vi "nD Line Search (VI).vi"(5 "J":dbl[][](array[numeric]) format="%.2f", 6 "data":variant, 7 "F(X)":T1, 8 "TOLX":dbl=1e-07 format="%.2e", 9 "alpha":dbl=0.0001 format="%.2e", 10 "P":dbl[](array[numeric]) format="%.2f", 11 "X":dbl[](array[numeric]) format="%.2f") -> (0 "error":i32, 2 "index":u32, 3 "X (new)":dbl[](array[numeric]) format="%.2f")   [LabVIEW 2010, in "NI_Gmath.lvlib"]
uses:
  NI_Gmath.lvlib
  functionRefnum nD.ctl
  Real Dot Product.vi
  NI_AALBase.lvlib
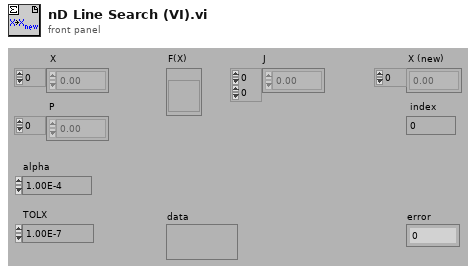
[diagram p1: front panel]
types:
  T1 = typedef "NI_Gmath.lvlib/functionRefnum nD.ctl" = refnum<vi>
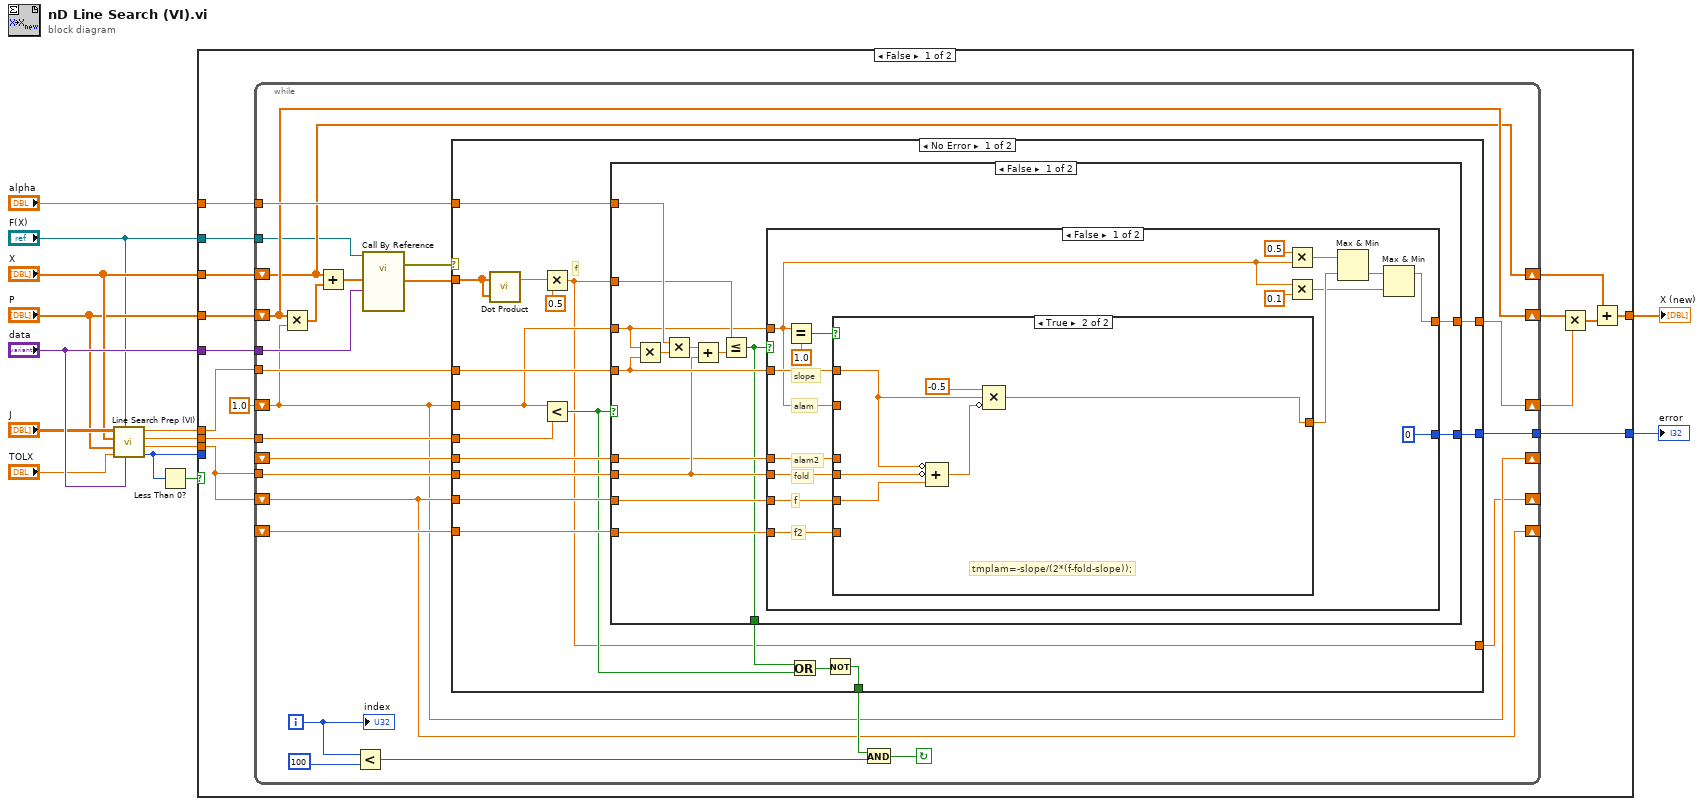
[diagram p0: block diagram]
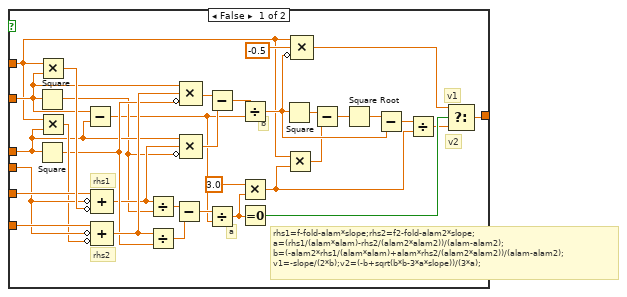
[diagram p2: hidden frame]
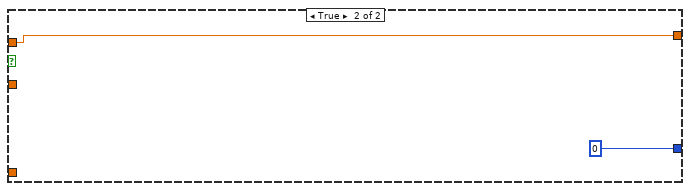
[diagram p3: hidden frame]
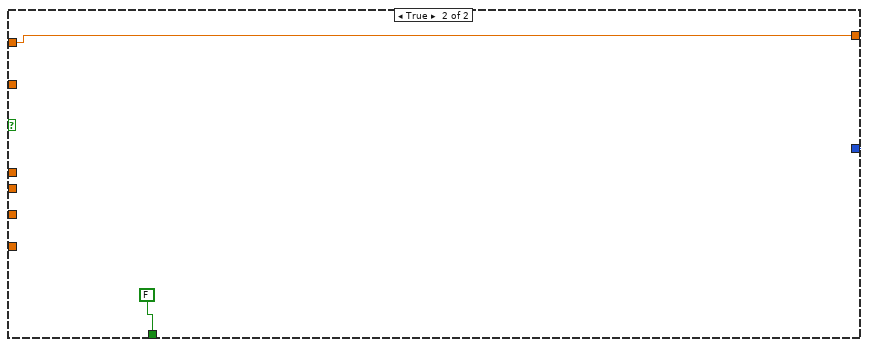
[diagram p4: hidden frame]
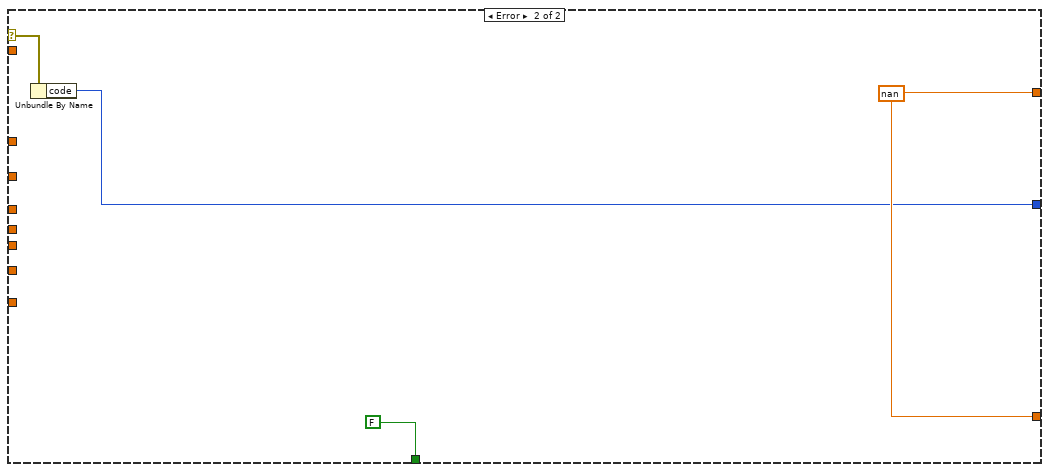
[diagram p5: hidden frame]
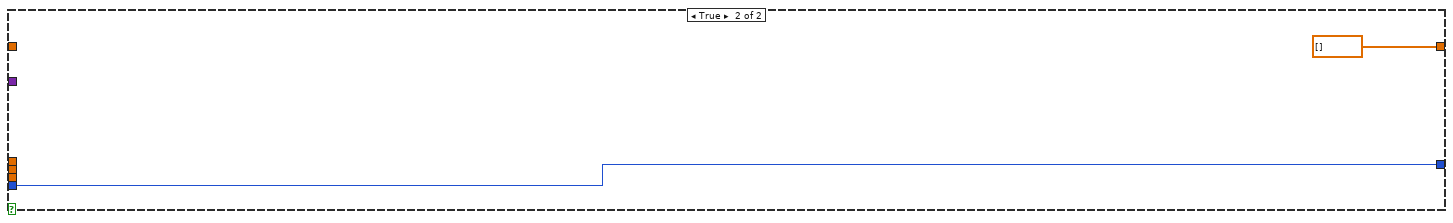
[diagram p6: hidden frame]
diagram:
  n1 = call "Line Search Prep (VI).vi"("data"="data", "F(X)"="F(X)", "TOLX"="TOLX", "P"="P", "X"="X", "J"="J") -> ("error"=w3:i32, "F(X)*F(X)"=w9:dbl, "tolerance"=w11:dbl, "X * Y"=w10:dbl)  [unwired: 2 out]
  n2 = Less Than 0?(x=w3) -> (x < 0?=w4:bool)
  n3 = case shown="False" w4 {
    tunnel: "data" -> [w29 _]
    tunnel: w11 -> [w27 _]
    tunnel: w10 -> [w26 _]
    tunnel: w9 -> [w25 _]
    tunnel: [w20 dbl[] []] -> w8
    tunnel: "alpha" -> [w19 _]
    tunnel: "X" -> [w18 _]
    tunnel: "P" -> [w17 _]
    tunnel: "F(X)" -> [w16 _]
    tunnel: w3 -> [_ w151]
    tunnel: [w15 w151] -> w2
    frame False {
      n4 = while {
        tunnel: w25 -> [w49]
        tunnel: w26 -> [w50]
        tunnel: w19 -> [w51]
        tunnel: w27 -> [w52]
        shift-left: _ -> [w48]
        shift-right: [w35] -> _
        shift-left: w25 -> [w35]
        shift-right: [w32] -> _
        shift-left: _ -> [w47]
        shift-right: [w34] -> _
        shift-left: 1.0 -> [w34]
        shift-right: [w43] -> w23
        shift-left: w17 -> [w46]
        shift-right: [w46] -> w22
        shift-left: w18 -> [w45]
        shift-right: [w45] -> w24
        tunnel: w16 -> [w38]
        tunnel: w29 -> [w37]
        tunnel: [w33] -> w15
        i -> [w44]
        stop <- w39 continue-if-true
        n5 = Multiply(x=w46, y=w34) -> (x*y=w53:dbl[])
        n6 = Add(x=w45, y=w53) -> (x+y=w31:dbl[])
        n7 = Less?(x=w44, y=100) -> (x < y?=w41:bool)
        n8 = call-by-ref "?"(reference=w38, "variant"=w37, "X"=w31) -> (error out=w30:errorcluster, "F(X)"=w36:dbl[])  [unwired: 4 in, 1 out]
        n9 = case shown="No Error" w30 {
          selector: w30 -> [_ w147]
          tunnel: w52 -> [w71 _]
          tunnel: w51 -> [w70 _]
          tunnel: w50 -> [w69 _]
          tunnel: w49 -> [w68 _]
          tunnel: w35 -> [w64 _]
          tunnel: w48 -> [w63 _]
          tunnel: w47 -> [w62 _]
          tunnel: [w59 w148] -> w43
          tunnel: [w58 FALSE] -> w40
          tunnel: w36 -> [w57 _]
          tunnel: w34 -> [w56 _]
          tunnel: [w55 w148] -> w32
          tunnel: [w54 w146] -> w33
          frame No Error {
            # "f"
            n10 = call-poly "Dot Product.vi"("Y Vector"=w57, "X Vector"=w57) -> ("X * Y"=w67:dbl)  [unwired: 1 out]
            n11 = Multiply(x=w67, y=0.5) -> (x*y=w55:dbl)
            n12 = Less?(x=w56, y=w71) -> (x < y?=w61:bool)
            n13 = case shown="False" w61 {
              tunnel: w70 -> [w85 _]
              tunnel: w56 -> [w80 w144]
              tunnel: w69 -> [w78 _]
              tunnel: w68 -> [w76 _]
              tunnel: w55 -> [w81 _]
              tunnel: [w73 FALSE] -> w65
              tunnel: [w79 w144] -> w59
              tunnel: w64 -> [w77 _]
              tunnel: w63 -> [w75 _]
              tunnel: w62 -> [w74 _]
              tunnel: [w72 0] -> w54
              frame False {
                n14 = Multiply(x=w80, y=w78) -> (x*y=w84:dbl)
                n15 = Multiply(x=w85, y=w84) -> (x*y=w83:dbl)
                n16 = Add(x=w83, y=w76) -> (x+y=w82:dbl)
                n17 = Less Or Equal?(x=w81, y=w82) -> (x <= y?=w73:bool)
                n18 = case shown="False" w73 {
                  tunnel: w80 -> [w89 w142]
                  tunnel: [w93 w142] -> w79
                  tunnel: w78 -> [w92 _]
                  tunnel: w77 -> [w91 _]
                  tunnel: w76 -> [w90 _]
                  tunnel: w75 -> [w88 _]
                  tunnel: w74 -> [w87 _]
                  tunnel: [0 0] -> w72
                  frame False {
                    # "f2"
                    # "f"
                    # "slope"
                    # "fold"
                    # "alam2"
                    # "alam"
                    n19 = Equal?(x=w89, y=1.0) -> (x = y?=w100:bool)
                    n20 = case shown="True" w100 {
                      tunnel: [w133 w138] -> w97
                      tunnel: w92 -> [w106 w135]
                      tunnel: w91 -> [w131 w137]
                      tunnel: w90 -> [w129 w136]
                      tunnel: w89 -> [w124 _]
                      tunnel: w88 -> [w130 _]
                      tunnel: w87 -> [w119 _]
                      frame False {
                        # "rhs1=f-fold-alam*slope;rhs2=f2-fold-alam2*slope;\na=(rhs1/(alam*alam)-rhs2/(alam2*alam2))/(alam-alam2);\nb=(-alam2*rhs1/(alam*alam)+alam*rhs2/(alam2*alam2))/(alam-alam2);\nv1=-slope/(2*b);v2=(-b+sqrt(b*b-3*a*slope))/(3*a);"
                        # "rhs2"
                        # "rhs1"
                        # "b"
                        # "v2"
                        # "v1"
                        # "a"
                        n21 = Square(x=w124) -> (x^2=w118:dbl)
                        n22 = Square(x=w119) -> (x^2=w122:dbl)
                        n23 = Multiply(x=w106, y=w124) -> (x*y=w132:dbl)
                        n24 = Multiply(x=w106, y=w119) -> (x*y=w128:dbl)
                        n25 = Subtract(x=w124, y=w119) -> (x-y=w115:dbl)
                        n26 = Compound Arithmetic op=ADD(w131, invert w129, invert w132) -> (w120:dbl)
                        n27 = Compound Arithmetic op=ADD(w130, invert w129, invert w128) -> (w123:dbl)
                        n28 = Divide(x=w120, y=w118) -> (x/y=w127:dbl)
                        n29 = Divide(x=w123, y=w122) -> (x/y=w126:dbl)
                        n30 = Subtract(x=w127, y=w126) -> (x-y=w125:dbl)
                        n31 = Compound Arithmetic op=MULTIPLY(w124, w123, invert w122) -> (w121:dbl)
                        n32 = Compound Arithmetic op=MULTIPLY(w119, w120, invert w118) -> (w117:dbl)
                        n33 = Subtract(x=w121, y=w117) -> (x-y=w116:dbl)
                        n34 = Divide(x=w125, y=w115) -> (x/y=w107:dbl)
                        n35 = Divide(x=w116, y=w115) -> (x/y=w109:dbl)
                        n36 = Multiply(x=3.0, y=w107) -> (x*y=w103:dbl)
                        n37 = Equal To 0?(x=w107) -> (x = 0?=w134:bool)
                        n38 = Square(x=w109) -> (x^2=w112:dbl)
                        n39 = Multiply(x=w106, y=w103) -> (x*y=w105:dbl)
                        n40 = Compound Arithmetic op=MULTIPLY(w106, -0.5, invert w109) -> (w113:dbl)
                        n41 = Subtract(x=w112, y=w105) -> (x-y=w111:dbl)
                        n42 = Square Root(x=w111) -> (sqrt(x)=w110:dbl)
                        n43 = Subtract(x=w110, y=w109) -> (x-y=w104:dbl)
                        n44 = Divide(x=w104, y=w103) -> (x/y=w102:dbl)
                        n45 = Select(t=w113, s=w134, f=w102) -> (s? t:f=w133:dbl)
                      }
                      frame True {
                        # "tmplam=-slope/(2*(f-fold-slope));"
                        n46 = Compound Arithmetic op=ADD(invert w135, invert w136, w137) -> (w140:dbl)
                        n47 = Compound Arithmetic op=MULTIPLY(-0.5, w135, invert w140) -> (w138:dbl)
                      }
                    }
                    n48 = Multiply(x=0.5, y=w89) -> (x*y=w98:dbl)
                    n49 = Multiply(x=w89, y=0.1) -> (x*y=w94:dbl)
                    n50 = Max & Min(x=w98, y=w97) -> (min(x,y)=w95:dbl)  [unwired: 1 out]
                    n51 = Max & Min(x=w95, y=w94) -> (max(x,y)=w93:dbl)  [unwired: 1 out]
                  }
                  frame True {
                  }
                }
              }
              frame True {
              }
            }
            n52 = Or(x=w65, y=w61) -> (x .or. y?=w60:bool)
            n53 = Not(x=w60) -> (.not. x?=w58:bool)
          }
          frame Error {
            w148 = nan
            n54 = Unbundle By Name(w147) -> ("code"=w146:i32)
          }
        }
        n55 = And(x=w40, y=w41) -> (x .and. y?=w39:bool)
        "index" <- w44
      }
      n56 = Multiply(x=w22, y=w23) -> (x*y=w21:dbl[])
      n57 = Add(x=w24, y=w21) -> (x+y=w20:dbl[])
    }
    frame True {
    }
  }
  "X (new)" <- w8
  "error" <- w2
